vi "e.gate HighSpeedPort Check Command Supported.vi"(8 "error in (no error)":errorcluster, 11 "Configuration in":T1) -> (0 "error out":errorcluster, 3 "Configuration out":T1)   [LabVIEW 2016]
doc: "This VI is used to check if HighSpeedPortBuffer Commands are supported by the connected controller.\n(ReadBufferSingleWithStateResponse in #summary.sta)"
uses:
  e.gate Configuration.ctl
  e.gate Channel Data.ctl
  e.gate Data Type.ctl
  e.gate Protocol Type.ctl
  e.gate Module  Data.ctl
  e.gateHSP_DLLhandle.ctl
  <vilib>/Utility/config.llb/Read Key (I32).vi
  <vilib>/Utility/config.llb/NI_LVConfig.lvlib
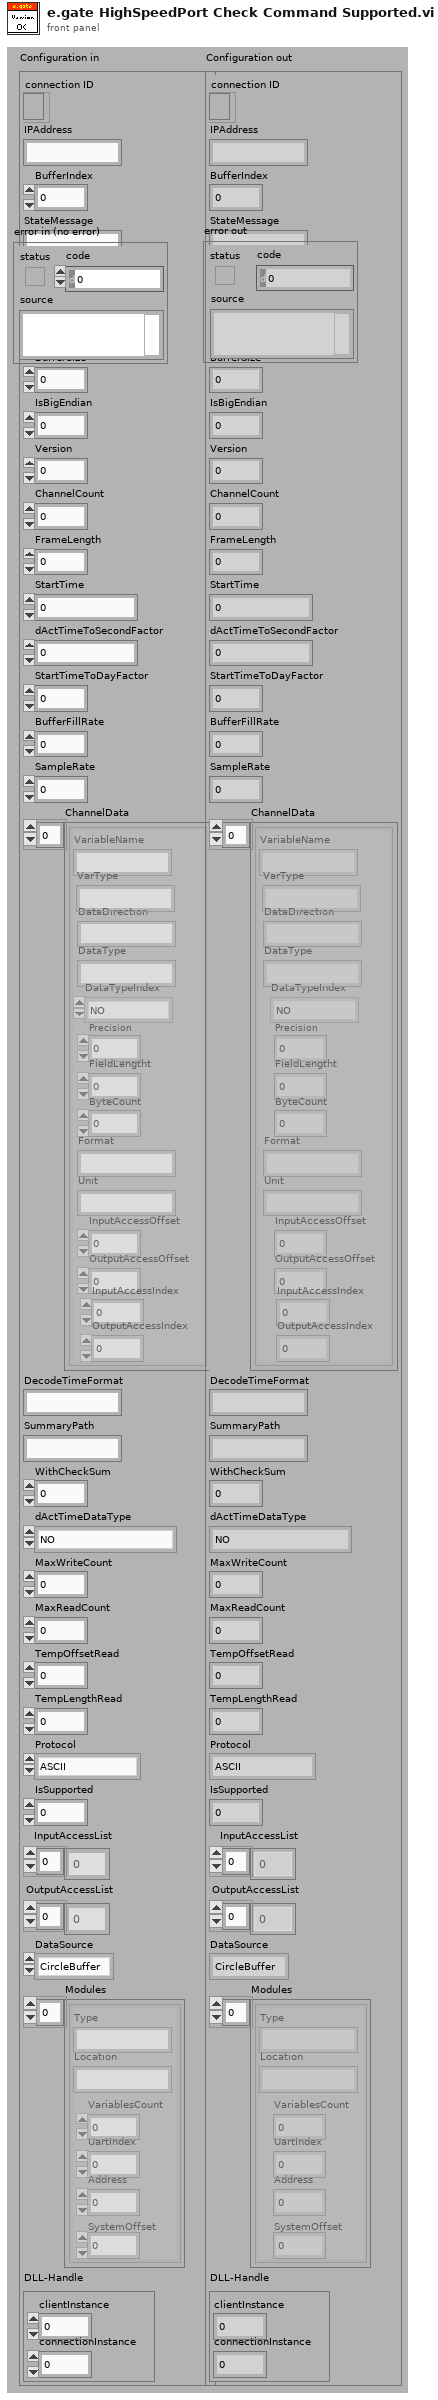
[diagram p1: front panel]
types:
  T1 = typedef "e.gate Configuration.ctl" = cluster{"connection ID":refnum<k5>, "IPAddress":string, "BufferIndex":i32, "StateMessage":string, "StateCode":i8, "HeaderSize":i32, "BufferSize":i32, "IsBigEndian":i32, "Version":i32, "ChannelCount":i32, "FrameLength":i32, "StartTime":dbl, "dActTimeToSecondFactor":dbl, "StartTimeToDayFactor":dbl, "BufferFillRate":dbl, "SampleRate":dbl, "ChannelData":T2[], "DecodeTimeFormat":string, "SummaryPath":string, "WithCheckSum":i32, "dActTimeDataType":T3, "MaxWriteCount":i32, "MaxReadCount":i32, "TempOffsetRead":i32, "TempLengthRead":i32, "Protocol":T4, "IsSupported":i32, "InputAccessList":i32[], "OutputAccessList":i32[], "DataSource":enum16{"CircleBuffer", "test.con Logger", "test.con Archive"}, "Modules":T5[], "DLL-Handle":T6}
  T2 = typedef "e.gate Channel Data.ctl" = cluster{"VariableName":string, "DataDirection":string, "DataType":string, "DataTypeIndex":T3, "Precision":i16, "FieldLengtht":i16, "ByteCount":i32, "Format":string, "Unit":string, "InputAccessOffset":i32, "OutputAccessOffset":i16, "InputAccessIndex":i16, "OutputAccessIndex":i16, "VarType":string}
  T3 = typedef "e.gate Data Type.ctl" = enum16{"NO", "BOOL", "SINT8", "USINT8", "SINT16", "USINT16", "SINT32", "USINT32", "FLOAT", "SET8", "SET16", "SET32", "DOUBLE", "SINT64", "USINT64", "SET64"}
  T4 = typedef "e.gate Protocol Type.ctl" = enum16{"ASCII", "HighspeedPort Online", "HighspeedPort Buffer", "eGateHighspeedPortDLL "}
  T5 = typedef "e.gate Module  Data.ctl" = cluster{"Type":string, "Location":string, "VariablesCount":i16, "UartIndex":i16, "Address":i16, "SystemOffset":i16}
  T6 = typedef "e.gateHSP_DLLhandle.ctl" = cluster{"clientInstance":i32, "connectionInstance":i32}
  T7 = typedef "NI_LVConfig.lvlib/Config Data RefNum.ctl" = refnum<k1>
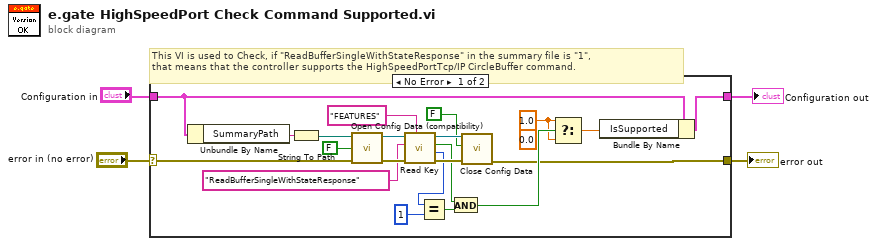
[diagram p0: block diagram]
diagram:
  # "This VI is used to Check, if \"ReadBufferSingleWithStateResponse\" in the summary file is \"1\",\nthat means that the controller supports the HighSpeedPortTcp/IP CircleBuffer command."
  n1 = case shown="No Error" "error in (no error)" {
    selector: "error in (no error)" -> [w18 w26]
    tunnel: [w6 w26] -> w1
    tunnel: [w7 w27] -> w3
    tunnel: "Configuration in" -> [w8 w27]
    frame No Error {
      (unwired) 0.0 ("f")
      w5 = 1.0 ("t")
      n2 = Unbundle By Name(w8) -> ("SummaryPath"=w25:string)
      n3 = String To Path(string=w25) -> (path=w24:path)
      n4 = call <vilib>:"Open Config Data (compatibility).vi"("error in (no error)"=w18, "create file if necessary (T)"=FALSE ("create file if necessary? (T)"), "configuration file path"=w24) -> ("error out"=w21:errorcluster, "refnum"=w23:T7)  [unwired: 6 in, 1 out]
      n5 = call-poly <vilib>:"Read Key.vi"("section"="FEATURES", "error in (no error)"=w21, "key"="ReadBufferSingleWithStateResponse", "refnum"=w23) -> ("error out"=w19:errorcluster, "value"=w12:i32, "found?"=w14:bool, "refnum out"=w20:T7)  [unwired: 1 in, 3 out]
      n6 = Equal?(x=w12, y=1) -> (x = y?=w13:bool)
      n7 = And(x=w14, y=w13) -> (x .and. y?=w10:bool)
      n8 = call <vilib>:"Close Config Data.vi"("error in (no error)"=w19, "write file if changed (T)"=FALSE ("write configuration file? (T)"), "refnum"=w20) -> ("error out"=w6:errorcluster)  [unwired: 8 out]
      n9 = Select(t=w5, s=w10, f=w5) -> (s? t:f=w9:dbl)
      n10 = Bundle By Name(cluster=w8, "IsSupported"=w9) -> (w7:T1)
    }
    frame Error {
    }
  }
  "Configuration out" <- w3
  "error out" <- w1
